vi "ReadAll(DBL).vi"(8 "错误输入":errorcluster) -> (0 "错误输出":errorcluster, 3 "TagDataArray":T1[](array[typedef]))   [LabVIEW 2013, in "Tag Data by Variant.lvlib"]
uses:
  Tag Data by Variant.lvlib
  Custom def/Tag DBL.ctl
  Custom def/mode.ctl
  Core/TagVar Data(DBL).vi
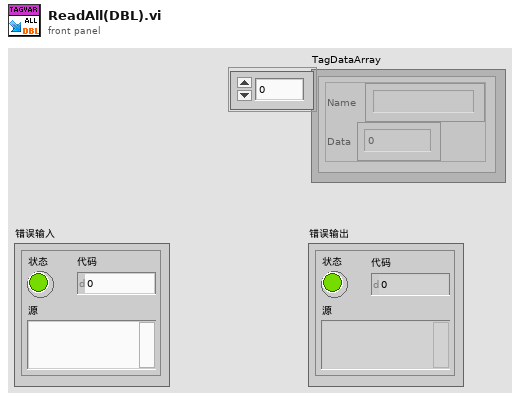
[diagram p1: front panel]
types:
  T1 = typedef "Tag Data by Variant.lvlib/Tag DBL.ctl" = cluster{"Name":string, "Data":dbl}
  T2 = typedef "Tag Data by Variant.lvlib/mode.ctl" = enum16{"初始化", "加入", "删除", "读取", "读取所有", "清除"}
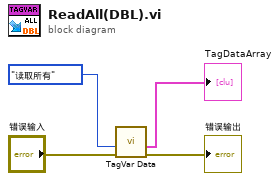
[diagram p0: block diagram]
diagram:
  n1 = call-poly "TagVar Data.vi"("错误输入"="错误输入", "method"=mode."读取所有") -> ("错误输出"=→"错误输出":errorcluster, "TagDataArray"=→"TagDataArray":T1[])  [unwired: 7 in, 1 out]
